vi "Arm Angle Calibrator.vi"() -> (1 "Voltage":dbl)   [LabVIEW 2013]
doc: "Analog Input Example\n\nThis example will read voltages from an analog channel and display it on a chart. It will also display the average voltage over time. \n\nThe values for Average Bits and Samples Per Second on the front panel can be set while the VI is running.\n\nThis example works with the NI 9201 module with an Analog Breakout attached. The Analog Breakout should have 12V applied to the WAGO connector (J3). Sensors are attached to the 3x8 header using 3-pin PWM connectors. The center pin of the 3-pin connector is 5V out that can be used to power sensors. The pin closest to the PCB (Printed Circuit Board) is ground. The pin farthest from the PCB is the signal input to be read by this VI. The signal range allowed is -10 volts to +10 volts."
panel:
  out "Angle":dbl
  in  "Sample Voltage":dbl=2.5
  in  "90 Voltage":dbl=1.67
  in  "180 Voltage":dbl=3.33
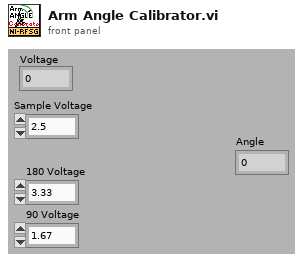
[diagram p1: front panel]
types:
  T1 = typedef "WPI_AnalogChannelDevRef.ctl" = cluster{"DevStatus":errorcluster, "Analog Module":T2, "Analog Channel":T3}
  T2 = typedef "FPGA_TypedefAnalogModule.ctl" = enum16{"Analog Module 1", "Analog Module 2"}
  T3 = typedef "FPGA_AIChannel.ctl" = enum8{"AI 1", "AI 2", "AI 3", "AI 4", "AI 5", "AI 6", "AI 7", "AI 8", "Invalid"}
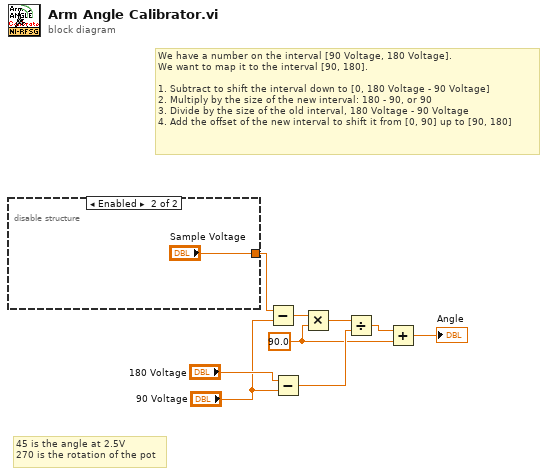
[diagram p0: block diagram]
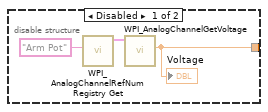
[diagram p2: hidden frame]
diagram:
  w2 = 90.0 ("y")
  # "We have a number on the interval [90 Voltage, 180 Voltage].\nWe want to map it to the interval [90, 180].\n\n1. Subtract to shift the interval down to [0, 180 Voltage - 90 Voltage]\n2. Multiply by the size of the new interval: 180 - 90, or 90\n3. Divide by the size of the old interval, 180 Voltage - 90 Voltage\n4. Add the offset of the new interval to shift it from [0, 90] up to [90, 180]"
  # "45 is the angle at 2.5V\n270 is the rotation of the pot"
  n1 = disable-structure shown="Enabled" {
    disable-tunnel: [w10 "Sample Voltage"] -> w9
    frame Disabled {
      n2 = call <vilib>:"WPI_AnalogChannelRefNum Registry Get.vi"("refnum name"="Arm Pot") -> ("AIDeviceRef"=w12:T1)  [unwired: 9 in, 1 out]
      n3 = call <vilib>:"WPI_AnalogChannelGetVoltage.vi"("AIDeviceRef"=w12) -> ("Voltage"=w10:dbl)  [unwired: 1 in, 9 out]
      "Voltage" <- w10
    }
    frame Enabled {
    }
  }
  n4 = Subtract(x=w9, y="90 Voltage") -> (x-y=w8:dbl)
  n5 = Subtract(x="180 Voltage", y="90 Voltage") -> (x-y=w4:dbl)
  n6 = Multiply(x=w8, y=w2) -> (x*y=w7:dbl)
  n7 = Divide(x=w7, y=w4) -> (x/y=w3:dbl)
  n8 = Add(x=w3, y=w2) -> (x+y=→"Angle":dbl)
